vi "fill-lstm-template.vi"() -> ()   [LabVIEW 2020]
uses:
  <vilib>/Analysis/7linalg.llb/Real Transpose Matrix.vi
  <vilib>/Analysis/Matrix/Numeric/Conversions/Array To Matrix - RA2.vi
  <vilib>/Analysis/Matrix/Numeric/Conversions/Matrix To Array - RM.vi
  <vilib>/Analysis/NI_AALPro.lvlib
  <vilib>/Analysis/Matrix/NI_Matrix.lvlib
panel:
  in  "weight path":path
  in  "name":string
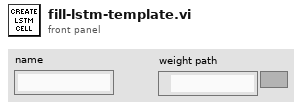
[diagram p1: front panel]
types:
  T1 = typedef "NI_Matrix.lvlib/RealMatrix.ctl" = dbl[][]
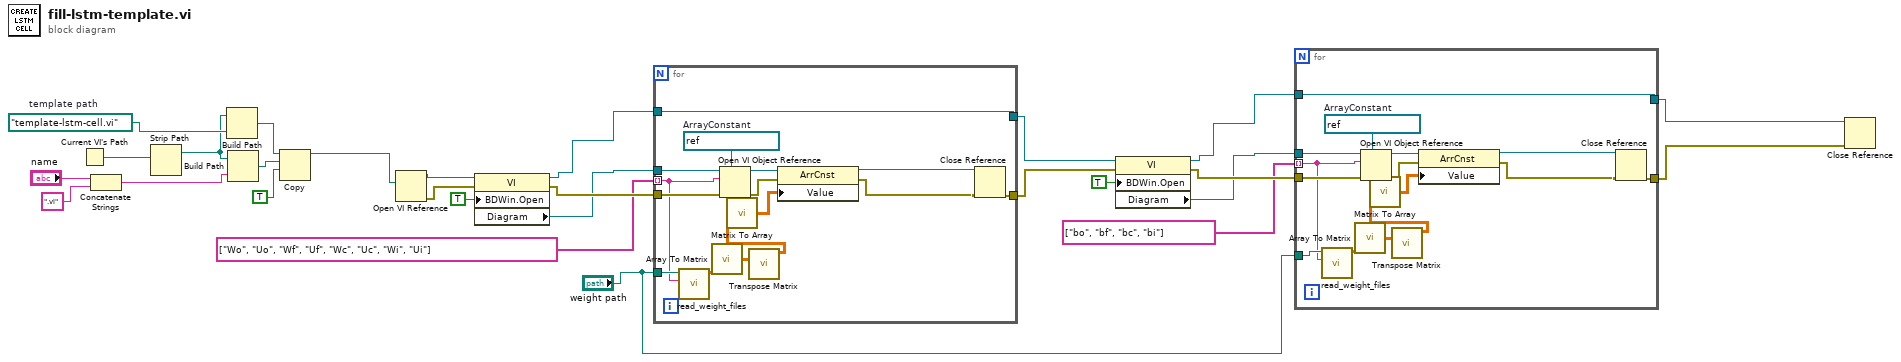
[diagram p0: block diagram]
diagram:
  w6 = path "template-lstm-cell.vi"  # template path
  n1 = Current VI's Path() -> (path=w5:path)
  n2 = Concatenate Strings("name", ".vi") -> (w7:string)
  n3 = Strip Path(path=w5) -> (stripped path=w4:path)  [unwired: 1 out]
  n4 = Build Path(base path=w4, name or relative path=w6) -> (appended path=w2:path)
  n5 = Build Path(base path=w4, name or relative path=w7) -> (appended path=w1:path)
  n6 = Copy(9:TRUE, 10:w1, 11:w2) -> (3:w22:path)  [unwired: 2 in, 2 out]
  n7 = Open VI Reference(vi path=w22) -> (vi reference=w24:refnum<vi>, error out=w23:errorcluster)  [unwired: 5 in]
  n8 = property class="VI"(reference=w24, error in=w23, "BDWin.Open"=TRUE) -> (reference out=w20:refnum<vi>, error out=w26:errorcluster, "Diagram"=w21:refnum<vi>)
  n9 = for {
    tunnel: w26 -> [w42]
    tunnel: w21 -> [w41]
    tunnel: string[] ["Wo", "Uo", "Wf", "Uf", "Wc", "Uc", "Wi", "Ui"] -> [w32] mode=indexing
    tunnel: [w36] -> w13
    tunnel: "weight path" -> [w33]
    tunnel: [w37] -> w14
    tunnel: w20 -> [w37]
    w40 = refnum<vi> refnum  # ArrayConstant
    n10 = call "read_weight_files.vi"("weight file name"=w32, "weights path"=w33) -> ("all rows"=w31:dbl[][])  [unwired: 9 in]
    n11 = call-poly <vilib>:"Array To Matrix.vi"("Real 2D Array"=w31) -> ("Real Matrix"=w30:T1)
    n12 = Open VI Object Reference(7:w40, 8:w42, 10:w32, 11:w41) -> (0:w38:errorcluster, 3:w39:refnum<vi>)
    n13 = call-poly <vilib>:"Transpose Matrix.vi"("Input Matrix"=w30) -> ("Matrix Transpose"=w29:T1)  [unwired: 9 in, 1 out]
    n14 = call-poly <vilib>:"Matrix To Array.vi"("Real Matrix"=w29) -> ("Real 2D Array"=w28:dbl[][])
    n15 = property class="ArrCnst"(reference=w39, error in=w38, "Value"=w28) -> (reference out=w35:refnum<vi>, error out=w34:errorcluster)
    n16 = Close Reference(reference=w35, error in (no error)=w34) -> (error out=w36:errorcluster)
  }
  n17 = property class="VI"(reference=w14, error in=w13, "BDWin.Open"=TRUE) -> (reference out=w15:refnum<vi>, error out=w17:errorcluster, "Diagram"=w16:refnum<vi>)
  n18 = for {
    tunnel: w17 -> [w57]
    tunnel: w16 -> [w56]
    tunnel: string[] ["bo", "bf", "bc", "bi"] -> [w44] mode=indexing
    tunnel: [w51] -> w10
    tunnel: "weight path" -> [w45]
    tunnel: [w52] -> w11
    tunnel: w15 -> [w52]
    w55 = refnum<vi> refnum  # ArrayConstant
    n19 = call "read_weight_files.vi"("weight file name"=w44, "weights path"=w45) -> ("all rows"=w48:dbl[][])  [unwired: 9 in]
    n20 = call-poly <vilib>:"Array To Matrix.vi"("Real 2D Array"=w48) -> ("Real Matrix"=w47:T1)
    n21 = Open VI Object Reference(7:w55, 8:w57, 10:w44, 11:w56) -> (0:w53:errorcluster, 3:w54:refnum<vi>)
    n22 = call-poly <vilib>:"Transpose Matrix.vi"("Input Matrix"=w47) -> ("Matrix Transpose"=w46:T1)  [unwired: 9 in, 1 out]
    n23 = call-poly <vilib>:"Matrix To Array.vi"("Real Matrix"=w46) -> ("Real 2D Array"=w43:dbl[][])
    n24 = property class="ArrCnst"(reference=w54, error in=w53, "Value"=w43) -> (reference out=w50:refnum<vi>, error out=w49:errorcluster)
    n25 = Close Reference(reference=w50, error in (no error)=w49) -> (error out=w51:errorcluster)
  }
  n26 = Close Reference(reference=w11, error in (no error)=w10) -> ()  [unwired: 1 out]
